vi "Time Into Trial.vi"(11 "Trial In Progress IN":bool) -> (3 "Time Into Trial (secs) OUT":dbl)   [LabVIEW 2018]
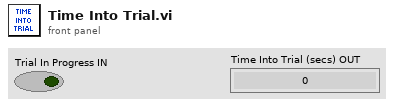
[diagram p1: front panel]
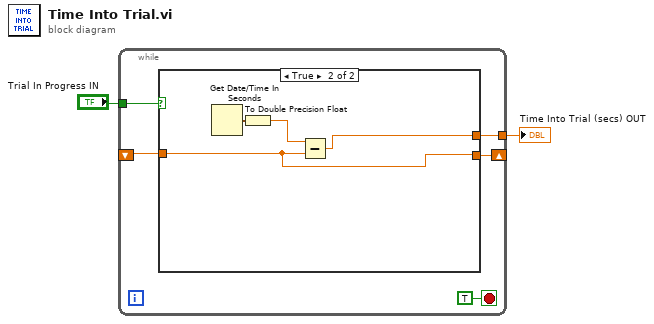
[diagram p0: block diagram]
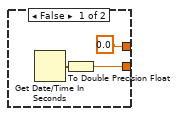
[diagram p2: hidden frame]
diagram:
  n1 = while {
    shift-right: [w6] -> _
    shift-left: _ -> [w5]
    tunnel: "Trial In Progress IN" -> [w4]
    tunnel: [w3] -> w1
    stop <- TRUE stop-if-true
    n2 = case shown="True" w4 {
      tunnel: [w9 w12] -> w6
      tunnel: w5 -> [_ w12]
      tunnel: [0.0 w11] -> w3
      frame False {
        n3 = Get Date/Time In Seconds() -> (seconds since 1Jan1904=w10:timestamp)
        n4 = To Double Precision Float(number=w10) -> (double precision float=w9:dbl)
      }
      frame True {
        n5 = Get Date/Time In Seconds() -> (seconds since 1Jan1904=w14:timestamp)
        n6 = To Double Precision Float(number=w14) -> (double precision float=w13:dbl)
        n7 = Subtract(x=w13, y=w12) -> (x-y=w11:dbl)
      }
    }
  }
  "Time Into Trial (secs) OUT" <- w1
